vi "Test_ConstructTransport_NoFormatString_NoError.vi"(8 "error in (no error)":errorcluster, 11 "TestCase in":refnum<class "TestBooleanTextBinding.lvclass">) -> (0 "error out":errorcluster, 3 "TestCase out":refnum<class "TestBooleanTextBinding.lvclass">)   [LabVIEW 2017, in "TestBooleanTextBinding.lvclass"]
uses:
  TestBooleanTextBinding.lvclass
  Source/Concrete/BooleanTextBinding/BooleanTextBinding.lvclass/BooleanTextBinding.ctl
  <vilib>/Utility/error.llb/Error Cluster From Error Code.vi
  Source/Concrete/BooleanTextBinding/BooleanTextBinding.lvclass
panel:
  in  "OK Button":bool
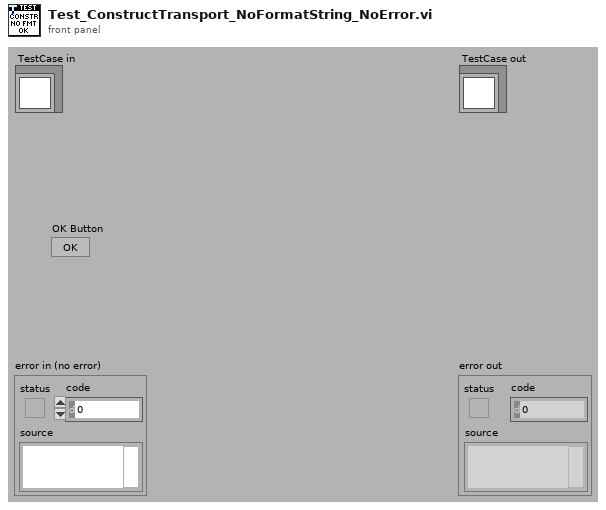
[diagram p1: front panel]
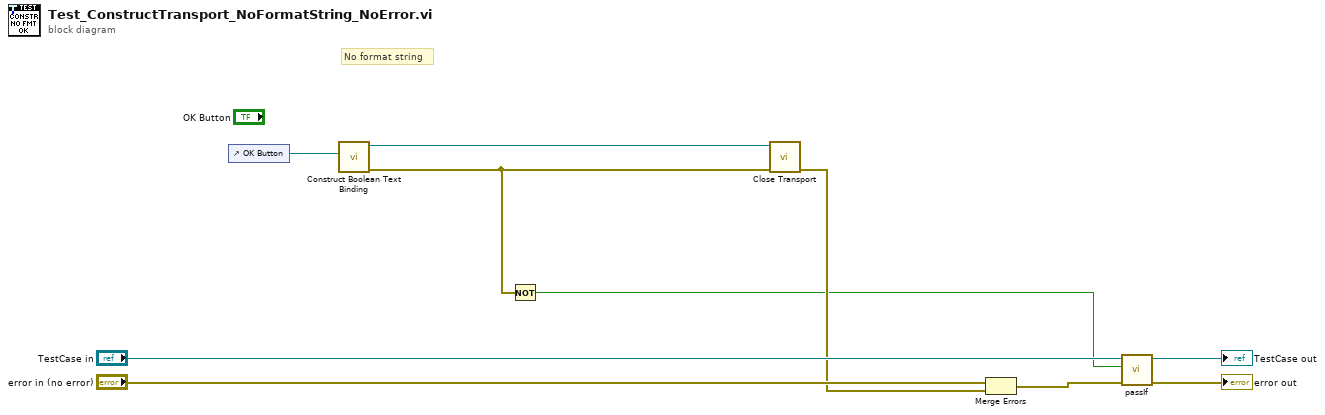
[diagram p0: block diagram]
diagram:
  # "No format string"
  n1 = control-ref of="OK Button"() -> (w5:refnum<vi>)
  n2 = call "Construct Boolean Text Binding.vi"("Bool Refnum"=w5) -> ("error out"=w2:errorcluster, "BooleanTextBinding"=w3:refnum<class "BooleanTextBinding.lvclass">)  [unwired: 9 in]
  n3 = Not(x=w2) -> (.not. x?=w1:bool)
  n4 = call-dynamic "Close Transport.vi"("error in (no error)"=w2, "ITransport in"=w3) -> ("error out"=w4:errorcluster)  [unwired: 9 in]
  n5 = Merge Errors("error in (no error)", w4) -> (w6:errorcluster)
  n6 = call-dynamic "passIf.vi"("error in (no error)"=w6, "pass"=w1, "TestCase in"="TestCase in") -> ("error out"=→"error out":errorcluster, "TestCase out"=→"TestCase out":refnum<class "TestBooleanTextBinding.lvclass">)  [unwired: 7 in]
